vi "GUI.vi"(8 "error in (no error)":errorcluster) -> (0 "error out":errorcluster)   [LabVIEW 2014]
uses:
  STD - Tap Mode.ctl
  Globals.vi
panel:
  in  "Quit Button":bool
  in  "Big Friendly Reset Button":bool
  out "Flappy Height Chart":cluster{"X":dbl, "Y":dbl}[](graph)
  out "Current Control Mode":T1
  out "Image height":i32
  out "Image width":i32
  in  "Play game!":bool
  in  "Image aligned?":bool
  out "Camera":T2(plugin-control)
  # "Use this if Flappy dies and you need to suspend the game\nIt will clear out whatever was planned\nFlappy will fall (if he was flying)\nAnd then it will return you to the start screen without starting"
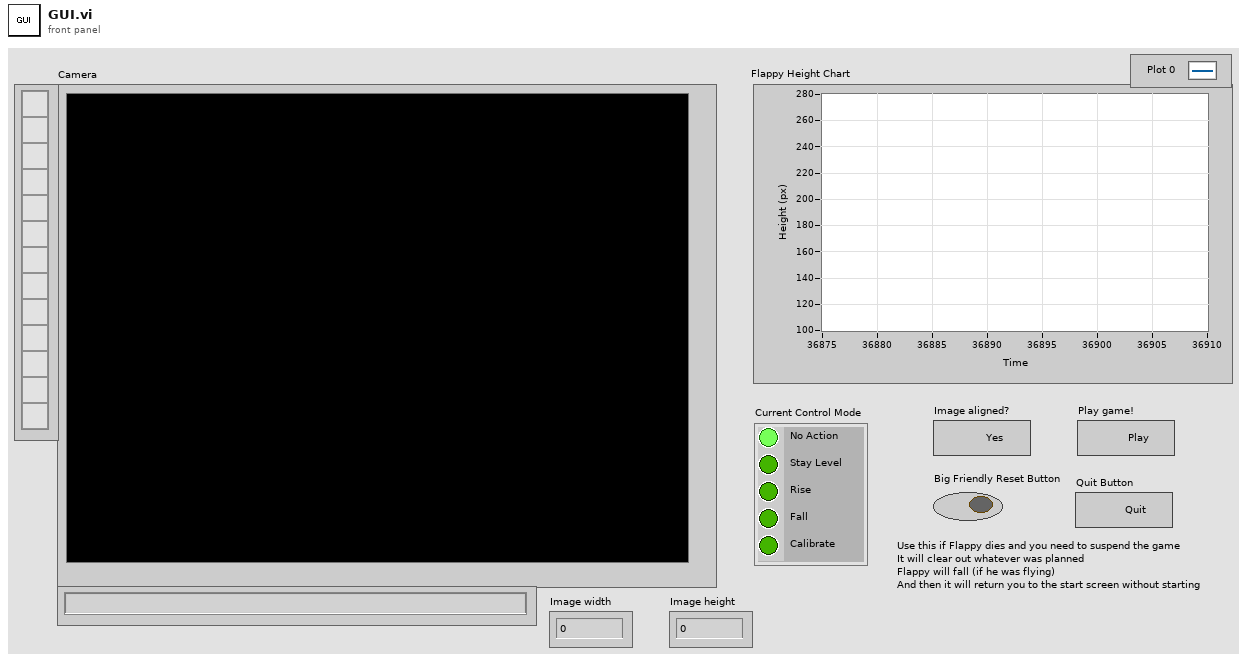
[diagram p1: front panel]
types:
  T1 = typedef "STD - Tap Mode.ctl" = enum32{"No Action", "Stay Level", "Rise", "Fall", "Calibrate"}
  T2 = typedef "IMAQ Image.ctl" = refnum<image>
  T3 = typedef "FlappyHeightPoint.ctl" = cluster{"Time (s)":dbl, "Height (px)":dbl}
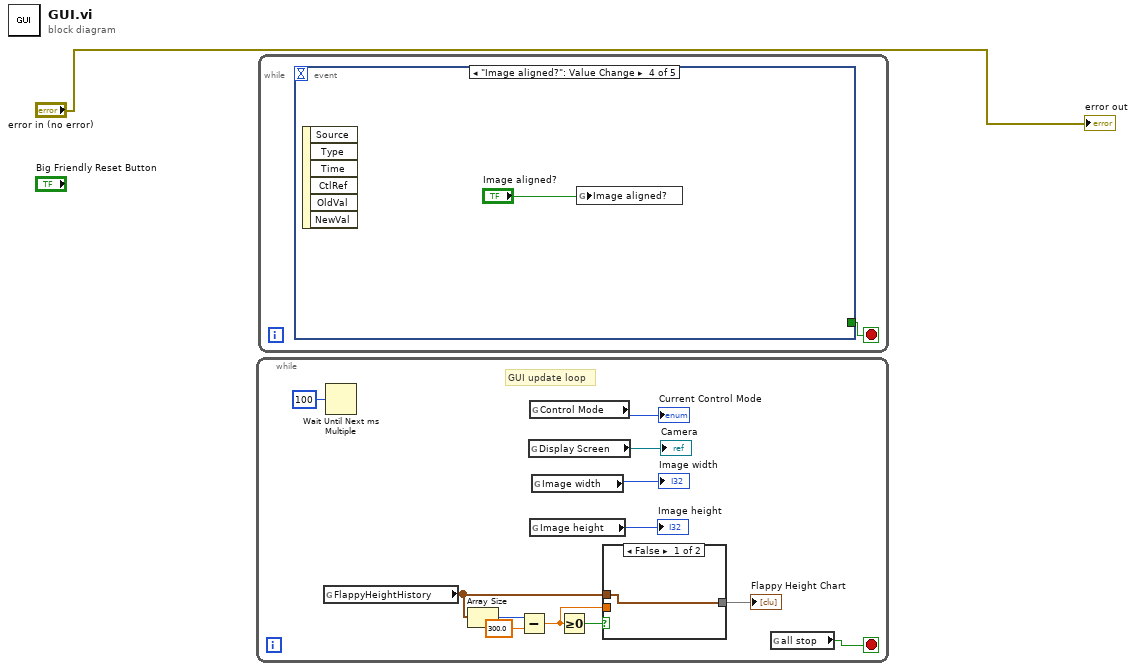
[diagram p0: block diagram]
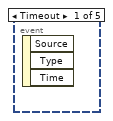
[diagram p2: hidden frame]
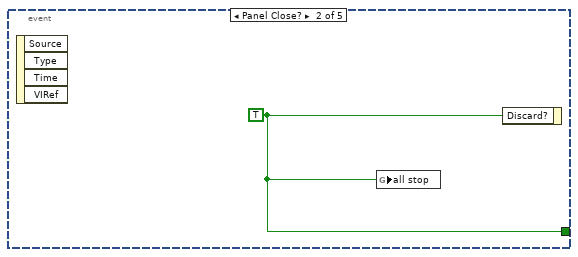
[diagram p3: hidden frame]
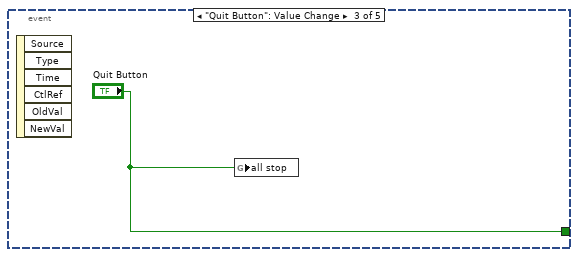
[diagram p4: hidden frame]
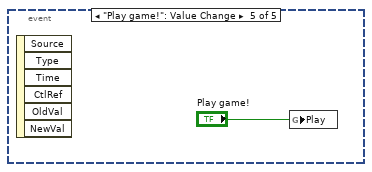
[diagram p5: hidden frame]
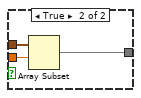
[diagram p6: hidden frame]
diagram:
  n1 = while {
    stop <- w2 stop-if-true
    # "GUI update loop"
    n2 = global read "Globals.vi" "FlappyHeightHistory"() -> (w7:T3[])
    n3 = Wait Until Next ms Multiple(millisecond multiple=u32 100) -> ()  [unwired: 1 out]
    n4 = Array Size(array=w7) -> (size(s)=w9:i32)
    n5 = Subtract(x=w9, y=300.0) -> (x-y=w8:dbl)
    n6 = global read "Globals.vi" "Display Screen"() -> (→"Camera":T2)
    n7 = global read "Globals.vi" "Control Mode"() -> (→"Current Control Mode":T1)
    n8 = global read "Globals.vi" "Image height"() -> (→"Image height":u32)
    n9 = global read "Globals.vi" "Image width"() -> (→"Image width":u32)
    n10 = Greater Or Equal To 0?(x=w8) -> (x >= 0?=w6:bool)
    n11 = case shown="False" w6 {
      tunnel: w8 -> [_ w17]
      tunnel: w7 -> [w14 w16]
      tunnel: [w14 w15] -> w5
      frame False {
      }
      frame True {
        n12 = Array Subset(array=w16, index=w17) -> (w15:T3[])  [unwired: 1 in]
      }
    }
    "Flappy Height Chart" <- w5
    n13 = global read "Globals.vi" "all stop"() -> (w2:bool)
  }
  n14 = while {
    stop <- w18 stop-if-true
    n15 = event shown="[3] \"Image aligned?\": Value Change" {
      selector: _ -> [_ _ _ _ _]
      dyn-events: _ -> [_ _ _ _ _]
      timeout: _ -> [_ _ _ _ _]
      tunnel: [_ w19 "Quit Button" _ _] -> w18
      event Timeout {
        n16 = event-data() -> ()  [unwired: 1 in, 3 out]
      }
      event Panel Close? {
        w19 = TRUE ("Discard?")
        n17 = event-data() -> ()  [unwired: 1 in, 4 out]
        n18 = global write "Globals.vi" "all stop"(w19) -> ()
        n19 = event-data("Discard?"=w19) -> ()  [unwired: 1 in, 1 out]
      }
      event "Quit Button": Value Change {
        n20 = event-data() -> ()  [unwired: 1 in, 6 out]
        n21 = global write "Globals.vi" "all stop"("Quit Button") -> ()
      }
      event "Image aligned?": Value Change {
        n22 = event-data() -> ()  [unwired: 1 in, 6 out]
        n23 = global write "Globals.vi" "Image aligned?"("Image aligned?") -> ()
      }
      event "Play game!": Value Change {
        n24 = event-data() -> ()  [unwired: 1 in, 6 out]
        n25 = global write "Globals.vi" "Play"("Play game!") -> ()
      }
    }
  }
  "error out" <- "error in (no error)"
